vi "Clusters and Bulndle exercise.vi"() -> ()   [LabVIEW 2024]
panel:
  out "array of clusters":cluster{"Boolean 3":bool}[](array[cluster])
  in  "Boolean 3":bool
  in  "Boolean 2":bool
  in  "Boolean":bool
  out "error out":errorcluster
  in  "error in (no error)":errorcluster
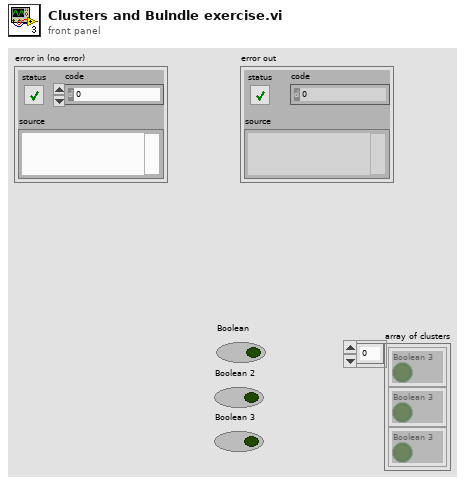
[diagram p1: front panel]
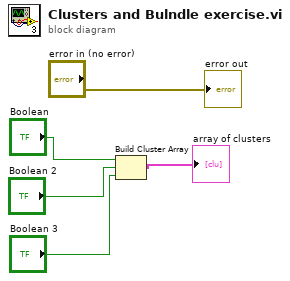
[diagram p0: block diagram]
diagram:
  n1 = Build Cluster Array("Boolean", "Boolean 2", "Boolean 3") -> (→"array of clusters":cluster{"Boolean 3":bool}[])
  "error out" <- "error in (no error)"
